vi "Stream Line On Axis Subset.vi"(5 "Symbolic Axes":string[](array[string]), 6 "Position Mode (0: absolute)":u16(ring) items=["absolute", "relative"], 7 "Coordinates":i64[](array[numeric]), 8 "error in (no error)":errorcluster, 9 "Device Number":string, 10 "Stream Number (1)":u8=1, 11 "VISA resource name":refnum<visa-resource-name>) -> (0 "error out":errorcluster, 3 "VISA resource name out":refnum<visa-resource-name>)   [LabVIEW 2015, in "Zaber A Series.lvlib"]
doc: "Adds a line command to an open stream, using a subset of the stream's axes. The line will always start where the previous stream command leaves the device positioned. The endpoint can be specified relative to there, or in absolute coordinates. The endpoint is specified in microstep units - use the Convert Position to Device Units VI to convert from standard measurements.\n\nThe Symbolic Axes input specifies which of the stream's axes the command will operate on. This can contain between one entry and the number of axes in the stream, and must have the same number of entries as the Coordinates input. The entries in the Symbolic Axes input are not axes numbers but letters that map to axes in the order the axes were added to the stream. For example, if the stream was set up with axes [1, 3, 2] then the symbol definitions will be a = 1, b = 3, c = 2. You can also permute the order in this input, so if you pass Symbolic Axes the input [c, b] in this example, then the coordinates you give will be for physical axes [2, 3].\n\nThis VI does not check in advance for error conditions such as streams not being supported or the stream not being open.\n\nThis VI requires that the device have Firmware version 7 and that the Initialize VI has been called with the same serial port and that the specified stream is open."
uses:
  Zaber A Series.lvlib
  Private/All Commands.ctl
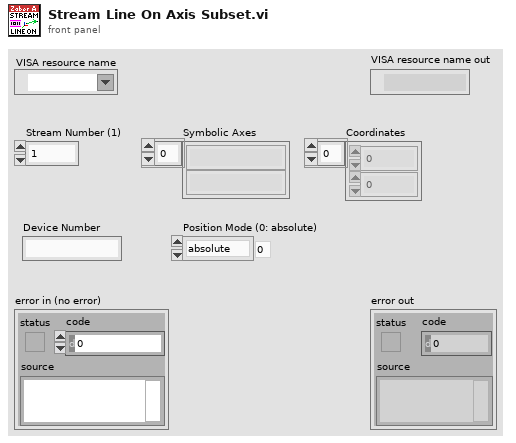
[diagram p1: front panel]
types:
  T1 = typedef "Zaber A Series.lvlib/All Commands.ctl" = string
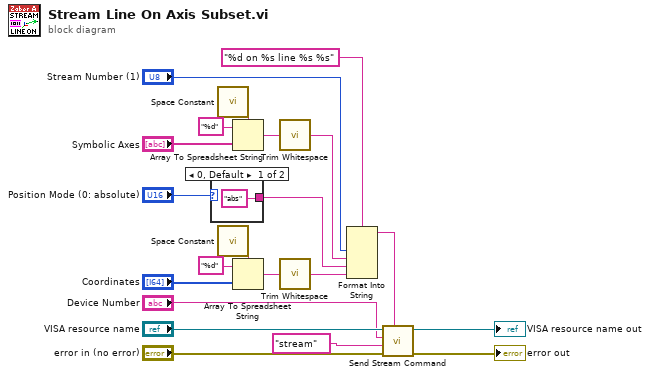
[diagram p0: block diagram]
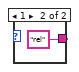
[diagram p2: hidden frame]
diagram:
  n1 = case shown="0, Default" "Position Mode (0: absolute)" {
    tunnel: ["abs" "rel"] -> w6
    frame 0, Default {
    }
    frame 1 {
    }
  }
  n2 = call <vilib>:"Space Constant.vi"() -> ("String"=w3:string)
  n3 = call <vilib>:"Space Constant.vi"() -> ("String"=w18:string)
  n4 = Array To Spreadsheet String(delimiter (Tab)=w3, array="Symbolic Axes", 3:"%d" ("format string")) -> (spreadsheet string=w2:string)
  n5 = Array To Spreadsheet String(delimiter (Tab)=w18, array="Coordinates", 3:"%d" ("format string")) -> (spreadsheet string=w12:string)
  n6 = call <vilib>:"Trim Whitespace.vi"("string"=w2) -> ("trimmed string"=w1:string)  [unwired: 1 in]
  n7 = call <vilib>:"Trim Whitespace.vi"("string"=w12) -> ("trimmed string"=w7:string)  [unwired: 1 in]
  n8 = Format Into String(format string="%d on %s line %s %s", "Stream Number (1)", w1, w6, w7) -> (resulting string=w9:string)  [unwired: 2 in, 1 out]
  n9 = call "Send Stream Command.vi"("Data"=w9, "error in (no error)"="error in (no error)", "Command"=T1 "stream" ("Complete Command List"), "Device Number"="Device Number", "VISA resource name"="VISA resource name") -> ("error out"=→"error out":errorcluster, "VISA resource name out"=→"VISA resource name out":refnum<visa-resource-name>)  [unwired: 5 in]
